vi "FestoCPX.Station.ProdLift.Ready.vi"(7 "Log (T)":bool=TRUE, 8 "error in":errorcluster, 10 "Position":T2, 11 "Slot":T1) -> (0 "error out":errorcluster, 2 "Ready state":T3)   [LabVIEW 2016]
uses:
  FestoCPX.Station.ProdLift.ReadyState.ctl
  Station/Station.ValvePosition.ctl
  Station/Station.ProductSlot.ctl
  tools/EventLog/EventLog.EventSource.ctl
  tools/Translator/Translator.Message.ctl
  tools/EventLog/EventLog.CreateError(single).vi
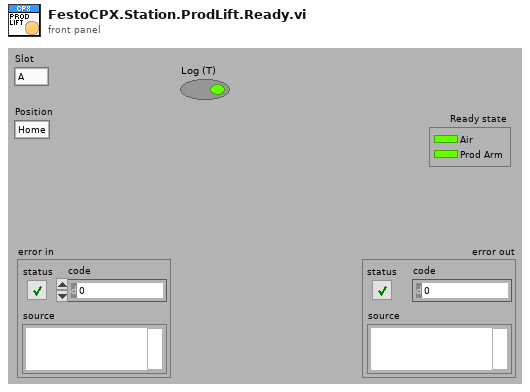
[diagram p1: front panel]
types:
  T1 = typedef "Station.ProductSlot.ctl" = enum8{"A", "B"}
  T2 = typedef "Station.ValvePosition.ctl" = enum16{"Home", "Work"}
  T3 = typedef "FestoCPX.Station.ProdLift.ReadyState.ctl" = cluster{"Air":bool, "Prod Arm":bool}
  T4 = typedef "EventLog.EventSource.ctl" = enum16{"All", "Gui", "Ref", "File", "Arch", "Seq", "CPX", "DB", "Laser", "Scan.P", "Scan.O"}
  T5 = typedef "Translator.Message.ctl" = enum16{"-", "Event confirmed", "Log out", "Log in", "Shutdown", "Cancel", "Start", "Begin time", "End time", "Duration", "Service Mode", "Ignore Results", "Serial Format", "On", "Off", "OK", "NOK", "NOK %s", "Home", "Work", "Close", "Open", "In progress...", "Missing", "Empty", "Hardware failure", "Initial", "Default", "Total", "Out of range", "Free disk space is below 1GB - contact technician", "Error %d >> %s", "Error %d >> %s >> %s", "Msg %d >> %s", "Laser msg %d %s", "Laser cmd error %s %d", "Laser cmd failed %s", "Laser cmd warning %s", "Laser disconnected", "Laser status %s", "Laser already started", "Laser job unkonwn %s", "Laser job missing %s", "Laser job select failure %s", "Unable to start laser printing (%s)", "Unable to stop laser printing (%s)", "Laser marking aborted", "Laser marking timeout", "Unable to reset Laser Interlock (%s)", "Unable to trigger Laser. Laser not ready (%s)", "Laser job '%s' coordinates not configured", "Starting %s", "Quitting %s", "Configured", "Initializing", "Quitting", "Loading", "Loaded %d results", "Loaded %d events", "Running", "Stopped", "Summary", "Laser", "Do you want to continue?", "Do you want to delete the configuration?", "The configuration is being used by an order. Unable to delete!", "Press confirm button", "Station is not based. Do you want to exit?", "Station requires changeover. Do you want to run the test?", "Test options are not set as default. Do you want to continue?", "Formatting of WabcoNo is disabled. Do you want to continue?", "Product not detected. Do you want to continue?", "Product scan failed. Do you want to continue?", "Calibration", "Log out?", "System", "All", "IDLE", "Translating...%s", "Not found", "Alarm %s", "Run", "Skip", "Abort", "Repeat", "Please wait...", "Database disconnected", "Database disconnected - changeover disabled!", "Login to database successful", "Login to database failed: %d; %s", "Unable to check the product status of reference %d - database disconnected", "Unable to set the product status of reference %d - database disconnected", "Variant file backup %s", "Read variant (%s)", "Result", "Station armed!", "Station requires changeover!", "Select reference number...", "EMERGENCY BUTTON - press Control button", "EMERGENCY DOOR - press Control button", "Resetting Emergency...", "Unable to reset safety circuit - Emergency Button pressed", "Unable to reset safety circuit - Emergency Side Door open", "Station not based", "Station based", "Station not empty", "Station basing...", "No order", "Press Start to begin new order", "Scanning new order", "Order NOK. Correct or scan again", "Order OK. Press Accept", "Order ready", "Revolver incorrect", "Fork incorrect", "Revolver missing", "Revolver empty", "Container missing", "Offline results", "Offline statistics", "Updating statistics %.1f %%", "DMC Configurator", "Door open", "Close the front door", "Press start button", "Done. Open the front door", "Running...", "Running...%.1f %%", "Pause %s", "Pause %s. NOK container missing", "Pause %s. OK container missing", "Pause %s. Revolver empty", "Pause %s. Revolver missing", "Pause %s. Revolver incorrect", "Pause %s. Fork missing", "Pause %s. Fork incorrect", "Pause %s. Too many failures", "Pause %s. Unloading failure", "Pause %s. One slot is not working", "Pause %s. Part order is done. Empty OK container", "Pause %s. Unable to move product to slot", "Pause %s. Unable to move back product pusher", "Pause %s. Unable to lift product", "Pause %s. Unable to move back product lifter", "Pause %s. Unable to move product arm to Work", "Pause %s. Unable to move product arm to NOK", "Pause %s. Unable to move product arm to OK", "Pause %s. Unable to unsuck the NOK product", "Pause %s. Unable to drop the NOK product", "Pause %s. Product OK missing", "Pause %s. Unable to unsuck the OK product", "Pause %s. Unable to drop the OK product", "Stopping...", "File '%s' is missing", "File '%s' is broken", "File '%s' is running", "Log file started (%s)", "Log file ended (%s)", "Log file stopped (%s)", "Log file ignored (%s)", "Log file exported (%s)", "Log file export failed (%s)", "Wrong serial number in log file", "Wrong reference number in log file", "Test steps are missing", "%s = %.3f", "Process param '%s' not found in DB", "Process param '%s' wrong order", "Process param '%s' value %.3f out of limits (%.3f; %.3f)", "Step%d param '%s' not found in DB", "Step%d param '%s' wrong order", "Step%d param '%s' value %.3f out of limits (%.3f; %.3f)", "Step%d EV '%s' not found in DB", "Step%d EV '%s' wrong order", "\"%s\" not found in DB", "\"%s\" wrong order", "\"%s\" value %.3f out of limits (%.3f; %.3f)", "\"%s\" not found in software", "Process init (%s)", "Process started", "Process restarted", "Process run", "Process done", "Process done - remove OK container", "Process aborted", "Process aborted at work", "Process aborted at home", "Process error", "Process error at home", "Process error at work", "Process close", "Process pause", "Process continue", "Process door open", "Process door close", "Process pause at slot %s due to %s", "Select plate from the order to process", "Do you want to start the process?", "Do you want to continue the process?", "There is unfinished order. Do you want to put the new order?", "Product %s %d OK", "Product %s %d NOK", "Unable to unload the slot %s. Product missing in the slot", "Unable to unload the slot %s. Product already in the arm", "Unable to accept the product as OK. Product missing in slot %s", "Unable to accept the product as OK. Product could not drop into the container at slot %s", "Unable to accept the product as NOK. Product could not drop into the container at slot %s", "Scan failed. Error %s", "Scan failed. Scanner disconnected", "Scan failed. Wrong Wabco number %d, limit (%d,%d)", "Scan failed. Wrong serial number %d, limit (%d,%d)", "Scan failed. Wrong date %d, limit (%d,%d)", "Scan failed. Wrong product wabco number %d (expected %d)", "Scan failed. Wrong product serial number %d (expected > 0)", "Scan OK %s", "Scan failed. Unable to determine table position (%s)", "Scan failed. Timeout", "Tune failed. Scanner disconnected", "Tune failed. Timeout", "%s = %d", "%s = %d->%d", "Unable to set %s = %.2f - Air Pressure Inside off", "Unable to set digital output '%s' = %d", "Unable to activate air pressure inside - timeout", "Unable to activate air pressure inside - aborted", "Unable to switch on Air Main Valve - Air Pressure Inlet off", "Unable to switch on Air Main Valve - Door open", "Unable to switch off Air Main Valve - timeout", "Unable to switch off Air Main Valve - aborted", "Unable to rotate Table - timeout", "Unable to rotate Table - aborted", "Unable to rotate Table - Product Move not in Home position", "Unable to rotate Table - Air Pressure Inside off", "Unable to rotate Table - Product Lift A not in Home position", "Unable to rotate Table - Product Lift B not in Home position", "Unable to rotate Table - unlock before movement timeout", "Unable to rotate Table - lock after movement timeout", "Unable to move Table Lock to %s position - timeout", "Unable to move Table Lock to %s position - aborted", "Unable to move Table Lock to %s position - Air Pressure Inside off", "Unable to move Table Lock to %s position - Table not in position", "Unable to move Product Lift A to %s position - timeout", "Unable to move Product Lift B to %s position - timeout", "Unable to move Product Lift A to %s position - aborted", "Unable to move Product Lift B to %s position - aborted", "Unable to move Product Lift A to %s position - Air Pressure Inside off", "Unable to move Product Lift B to %s position - Air Pressure Inside off", "Unable to move Product Lift A to %s position - Table not locked", "Unable to move Product Lift B to %s position - Table not locked", "Unable to move Product Lift A to %s position - Product Arm not in Work position", "Unable to move Product Lift B to %s position - Product Arm not in Work position", "Unable to set Product Suction Gripper %s to %s - timeout", "Unable to set Product Suction Gripper %s to %s - aborted", "Unable to set Product Suction Gripper %s to %s - Air Pressure Inside off", "Unable to set Product Suction Gripper %s to %s - Table slot unkown", "Unable to move Product Arm to %s position - timeout", "Unable to move Product Arm to %s position - aborted", "Unable to move Product Arm to %s position - Air Pressure Inside off", "Unable to move Product Arm to %s position - Product Lift A not in Home position", "Unable to move Product Arm to %s position - Product Lift B not in Home position", "Unable to move Product to %s position - timeout", "Unable to move Product to %s position - aborted", "Unable to move Product to %s position - Air Pressure Inside off", "Unable to move Product to %s position - Table not in position"}
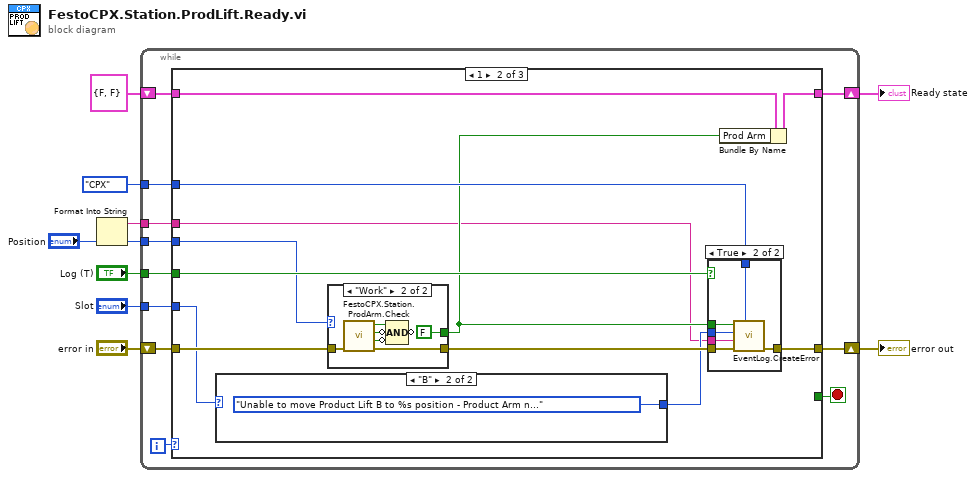
[diagram p0: block diagram]
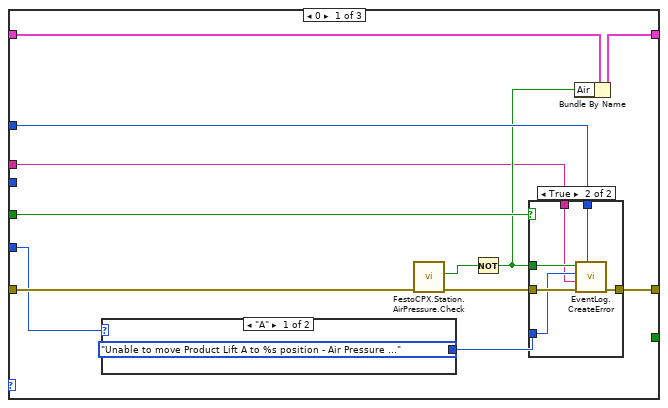
[diagram p2: hidden frame]
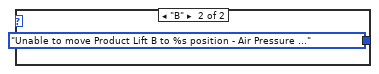
[diagram p3: hidden frame]
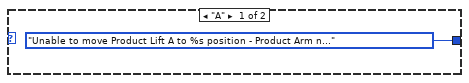
[diagram p6: hidden frame]
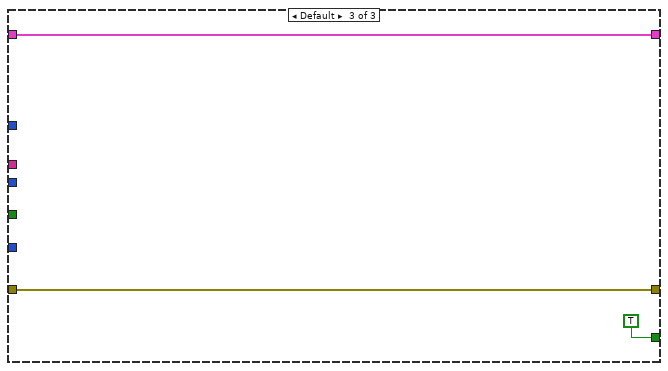
[diagram p8: hidden frame]
diagram:
  n1 = Format Into String("Position") -> (resulting string=w2:string)  [unwired: 3 in, 1 out]
  n2 = while {
    tunnel: "Log (T)" -> [w19]
    tunnel: EventLog.EventSource."CPX" ("Source") -> [w18]
    shift-right: [w13] -> w6
    shift-left: "error in" -> [w20]
    shift-right: [w14] -> w4
    shift-left: T3 {"Air"=FALSE, "Prod Arm"=FALSE} ("Ready state") -> [w15]
    tunnel: "Position" -> [w12]
    tunnel: w2 -> [w11]
    tunnel: "Slot" -> [w10]
    i -> [w17]
    stop <- w16 stop-if-true
    n3 = case shown="1" w17 {
      tunnel: w20 -> [w25 w50 w71]
      tunnel: [w27 w52 w70] -> w14
      tunnel: w19 -> [w26 w49 _]
      tunnel: w18 -> [w29 w47 _]
      tunnel: [_ _ TRUE] -> w16
      tunnel: w15 -> [w28 w53 w70]
      tunnel: [w30 w48 w71] -> w13
      tunnel: w12 -> [_ w42 _]
      tunnel: w11 -> [w22 w44 _]
      tunnel: w10 -> [w21 w43 _]
      frame 0 {
        n4 = case shown="\"A\"" w21 {
          tunnel: [Translator.Message."Unable to move Product Lift A to %s position - Air Pressure Inside off" ("msg") Translator.Message."Unable to move Product Lift B to %s position - Air Pressure Inside off" ("msg")] -> w31
          frame "A" {
          }
          frame "B" {
          }
        }
        n5 = call "FestoCPX.Station.AirPressure.Check.vi"("error in"=w25) -> ("error out"=w32:errorcluster, "Air pressure Inside"=w23:bool)  [unwired: 7 in, 2 out]
        n6 = Not(x=w23) -> (.not. x?=w24:bool)
        n7 = case shown="True" w26 {
          tunnel: w29 -> [_ w41]
          tunnel: w24 -> [_ w40]
          tunnel: w32 -> [w35 w39]
          tunnel: w31 -> [_ w38]
          tunnel: [w35 w37] -> w30
          tunnel: w22 -> [_ w36]
          frame False {
          }
          frame True {
            n8 = call-poly "EventLog.CreateError.vi"("Source (All)"=w41, "error in"=w39, "arg"=w36, "msg"=w38, "create (T)"=w40) -> ("error out"=w37:errorcluster)  [unwired: 6 in]
          }
        }
        n9 = Bundle By Name(cluster=w28, "Air"=w24) -> (w27:T3)
      }
      frame 1 {
        n10 = case shown="\"B\"" w43 {
          tunnel: [Translator.Message."Unable to move Product Lift A to %s position - Product Arm not in Work position" ("msg") Translator.Message."Unable to move Product Lift B to %s position - Product Arm not in Work position" ("msg")] -> w46
          frame "A" {
          }
          frame "B" {
          }
        }
        n11 = case shown="\"Work\"" w42 {
          tunnel: [w54 w60] -> w51
          tunnel: w50 -> [w54 w59]
          tunnel: [_ FALSE] -> w45
          frame "Home" {
          }
          frame "Work" {
            n12 = call "FestoCPX.Station.ProdArm.Check.vi"("error in"=w59) -> ("error out"=w60:errorcluster, "NOK"=w56:bool, "OK"=w57:bool, "Work"=w58:bool)  [unwired: 6 in, 1 out]
            n13 = Compound Arithmetic op=AND(w58, invert w57, invert w56) -> ()  [unwired: 1 out]
          }
        }
        n14 = case shown="True" w49 {
          tunnel: w47 -> [_ w69]
          tunnel: w45 -> [_ w68]
          tunnel: w51 -> [w63 w67]
          tunnel: w46 -> [_ w66]
          tunnel: [w63 w65] -> w48
          tunnel: w44 -> [_ w64]
          frame False {
          }
          frame True {
            n15 = call-poly "EventLog.CreateError.vi"("Source (All)"=w69, "error in"=w67, "arg"=w64, "msg"=w66, "create (T)"=w68) -> ("error out"=w65:errorcluster)  [unwired: 6 in]
          }
        }
        n16 = Bundle By Name(cluster=w53, "Prod Arm"=w45) -> (w52:T3)
      }
      frame Default {
      }
    }
  }
  "error out" <- w6
  "Ready state" <- w4
